vi "Global_TEC Monitor Loop_Status.vi"() -> ()   [LabVIEW 2019]
panel:
  in  "Reset":bool
  in  "Monitoring Active?":bool
  in  "Error":bool
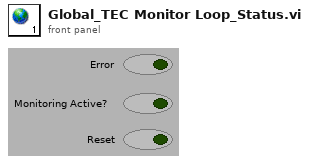
[diagram p1: front panel]
diagram:
